vi "ztscopeM Close.vi"(8 "error in":errorcluster, 11 "Instrument Handle In":i32) -> (0 "error out":errorcluster)   [LabVIEW 2013]
doc: "Close the passed in communication session. This does not affect other communication sessions that may have been opened."
uses:
  ztscopeM.dll
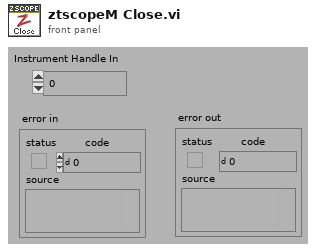
[diagram p1: front panel]
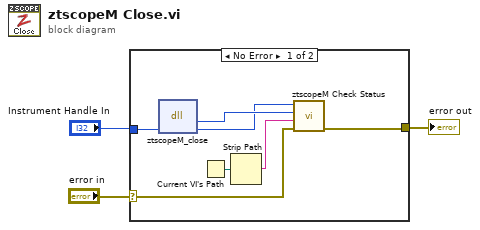
[diagram p0: block diagram]
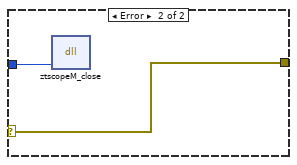
[diagram p2: hidden frame]
diagram:
  n1 = case shown="No Error" "error in" {
    selector: "error in" -> [w7 w12]
    tunnel: [w4 w12] -> w1
    tunnel: "Instrument Handle In" -> [w10 w11]
    frame No Error {
      n2 = dll-call lib="C:/Program Files/National Instruments/instr.lib/ztscopem/ztscopeM.dll" fn="ztscopeM_close"("instrumentHandle"=w10) -> (w6:i32, "instrumentHandle"=w5:i32)  [unwired: 3 in, 2 out]
      n3 = Current VI's Path() -> (path=w9:path)
      n4 = Strip Path(path=w9) -> (name=w8:string)  [unwired: 1 out]
      n5 = call "ztscopeM Check Status.vi"("error in"=w7, "name of VI"=w8, "status"=w6, "instrument handle in"=w5) -> ("error out"=w4:errorcluster)  [unwired: 2 in, 1 out]
    }
    frame Error {
      n6 = dll-call lib="C:/Program Files/National Instruments/instr.lib/ztscopem/ztscopeM.dll" fn="ztscopeM_close"("instrumentHandle"=w11) -> ()  [unwired: 5 in, 2 out]
    }
  }
  "error out" <- w1
